vi "practice-10-10.vi"() -> ()   [LabVIEW 2016]
uses:
  EFD Ultimus V/EFD Ultimus V.lvlib
panel:
  in  "Boolean":bool=TRUE
  in  "Numeric":i32
  in  "Serial Configuration":T1={"Baud Rate "=115200, "Parity "=0, "Data Bits "=8, "Stop Bits"=10} {"Stop Bits" items=["1.0"=10, "1.5"=15, "2.0"=20]; "Data Bits" items=["7"=7, "8"=8]; "Parity" items=["None", "Odd", "Even"]; "Baud Rate" items=["9600"=9600, "19200"=19200, "38400"=38400, "115200"=115200]}
  in  "VISA resource name":refnum<visa-resource-name>="COM5"
  in  "stop":bool
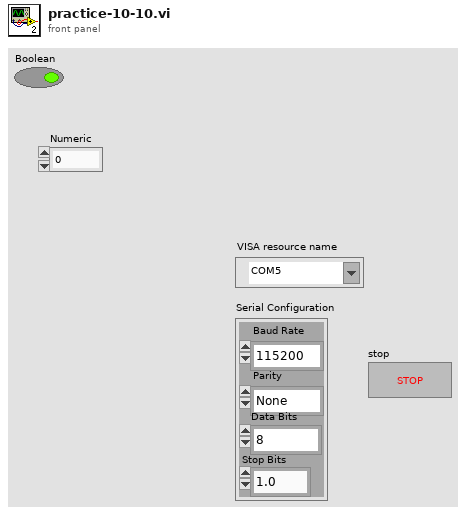
[diagram p1: front panel]
types:
  T1 = cluster{"Baud Rate ":u32, "Parity ":u16, "Data Bits ":u16, "Stop Bits":u16}
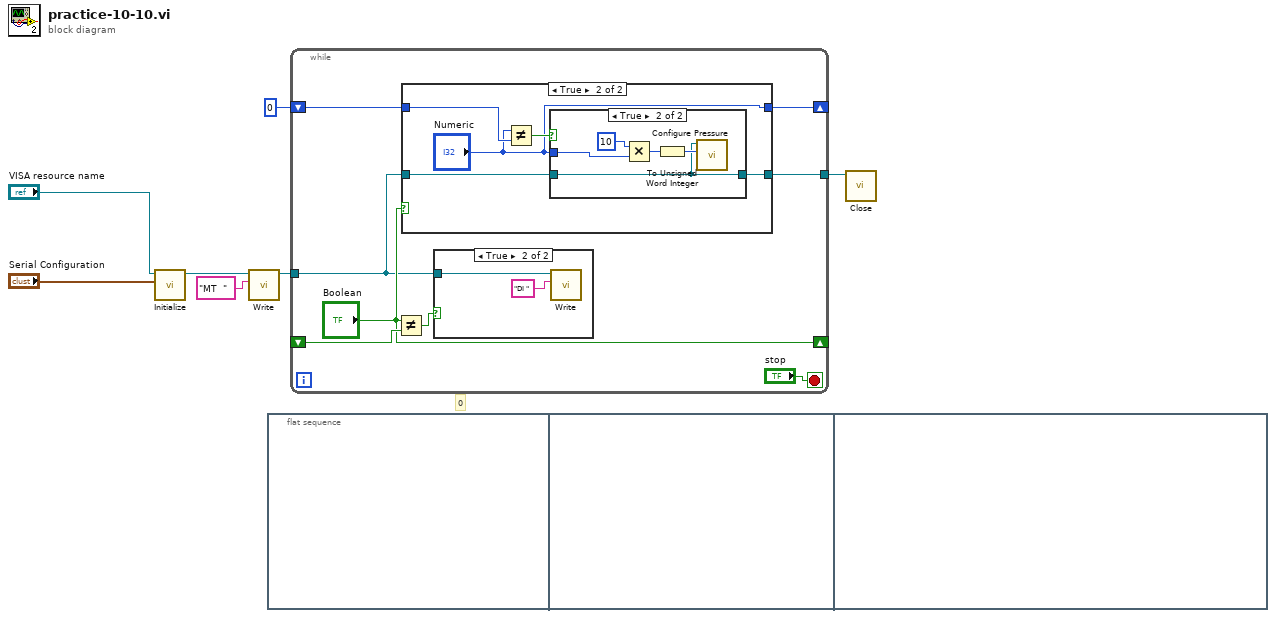
[diagram p0: block diagram]
diagram:
  # "0"
  n1 = call "Initialize.vi"("Serial Configuration"="Serial Configuration", "VISA resource name"="VISA resource name") -> ("VISA resource name out"=w5:refnum<visa-resource-name>)  [unwired: 8 in, 1 out]
  n2 = call "Write.vi"("Command To Write"="MT  ", "VISA resource name"=w5) -> ("VISA resource name out"=w3:refnum<visa-resource-name>)  [unwired: 8 in, 1 out]
  n3 = flat-sequence {
    frame #0 {
    }
    frame #1 {
    }
    frame #2 {
    }
  }
  n4 = while {
    tunnel: w3 -> [w8]
    tunnel: [w14] -> w2
    shift-right: [w12] -> _
    shift-left: 0 -> [w13]
    shift-right: ["Boolean"] -> _
    shift-left: _ -> [w11]
    stop <- "stop" stop-if-true
    n5 = Not Equal?(x="Boolean", y=w11) -> (x != y?=w9:bool)
    n6 = case shown="True" "Boolean" {
      tunnel: w8 -> [w19 w20]
      tunnel: [w19 w24] -> w14
      tunnel: w13 -> [w18 w23]
      tunnel: [w18 "Numeric"] -> w12
      frame False {
      }
      frame True {
        n7 = Not Equal?(x="Numeric", y=w23) -> (x != y?=w22:bool)
        n8 = case shown="True" w22 {
          tunnel: w20 -> [w25 w28]
          tunnel: [w25 w28] -> w24
          tunnel: "Numeric" -> [_ w27]
          frame False {
          }
          frame True {
            n9 = Multiply(x=10, y=w27) -> (x*y=w26:i32)
            n10 = To Unsigned Word Integer(number=w26) -> (unsigned 16bit integer=w29:u16)
            n11 = call "Configure Pressure.vi"("Pressure Setting (0000)"=w29, "VISA resource name"=w28) -> ()  [unwired: 8 in, 2 out]
          }
        }
      }
    }
    n12 = case shown="True" w9 {
      tunnel: w8 -> [_ w16]
      frame False {
      }
      frame True {
        n13 = call "Write.vi"("Command To Write"="DI ", "VISA resource name"=w16) -> ()  [unwired: 8 in, 2 out]
      }
    }
  }
  n14 = call "Close.vi"("VISA resource name"=w2) -> ()  [unwired: 10 in, 1 out]
